vi "Set Items.vi"(8 "error in (no error)":errorcluster, 10 "Items":refnum<class "IObject.lvclass">[](array[class]), 11 "IContainer in":refnum<class "IContainer.lvclass">) -> (0 "error out":errorcluster, 3 "IContainer out":refnum<class "IContainer.lvclass">)   [LabVIEW 2013, in "IContainer.lvclass"]
doc: "Copyright 2018, Wiebe Walstra, wiebe@carya.nl."
uses:
  IContainer.lvclass
  IObject.lvclass
  IContainer.lvclass/IContainer.ctl
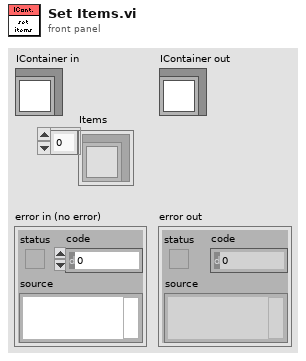
[diagram p1: front panel]
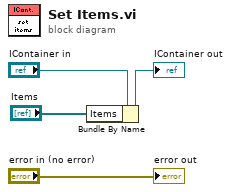
[diagram p0: block diagram]
diagram:
  n1 = Bundle By Name(cluster="IContainer in", "Items"="Items") -> (→"IContainer out":refnum<class "IContainer.lvclass">)
  "error out" <- "error in (no error)"
